vi "build.stepElement.vi"(11 "Step in":T1) -> (0 "error out":errorcluster, 3 "steps out":variant[](array[variant])=[variant("stepDoutString"=variant(string ""), "stepFunction"=variant(enum16{"__NO-OP", "_DELAY_LOAD", "_DELAY_COMPARE", "_COMPARE", "_JUMP", "_FINISH", "CLK_COMPARE", "PROC_START", "PROC_STOP", "PROC_ISRUN_IF_OFF", "PROC_ISRUN_LOAD", "_IO_READ_IN", "_IO_WRITE_DOUT", "_IO_COMPARE", "Q_OPEN", "Q_WRITE", "Q_READ"} enum."_IO_WRITE_DOUT"), "stepIoPointer"=variant(string ""), "stepLabel"=variant(string ""), "stepPath"=variant(string ""))])   [LabVIEW 2024]
uses:
  controls/UiStepBuilder.ctl
  controls/type.step-builder.ctl
  Polymorphics/variantCtrlStepFunction.vi
  Polymorphics/variantCtrlSetpoint.vi
  Polymorphics/variantCtrlString.vi
  util.DelimitedStringFromArray.vi
  Polymorphics/variantCtrlNumber.vi
  util.DelimitedStringToArray.vi
  proc.util.validateParamExist.vi
  <vilib>/Utility/error.llb/Clear Errors.vi
  <vilib>/Utility/error.llb/Trim Whitespace.vi
  <vilib>/Utility/error.llb/Trim Whitespace One-Sided.vi
  build.elementToParamString.vi
  util.error.create.vi
  Polymorphics/variantCtrlStepPointer.vi
  Polymorphics/variantCtrlStepUserMessage.vi
  Polymorphics/variantCtrlStepPath.vi
  controls/typeStepVarients.ctl
  controls/type.StepFunction.ctl
  <vilib>/Utility/miscctls.llb/LVPointTypeDef.ctl
panel:
  out "Step Argument Names":string
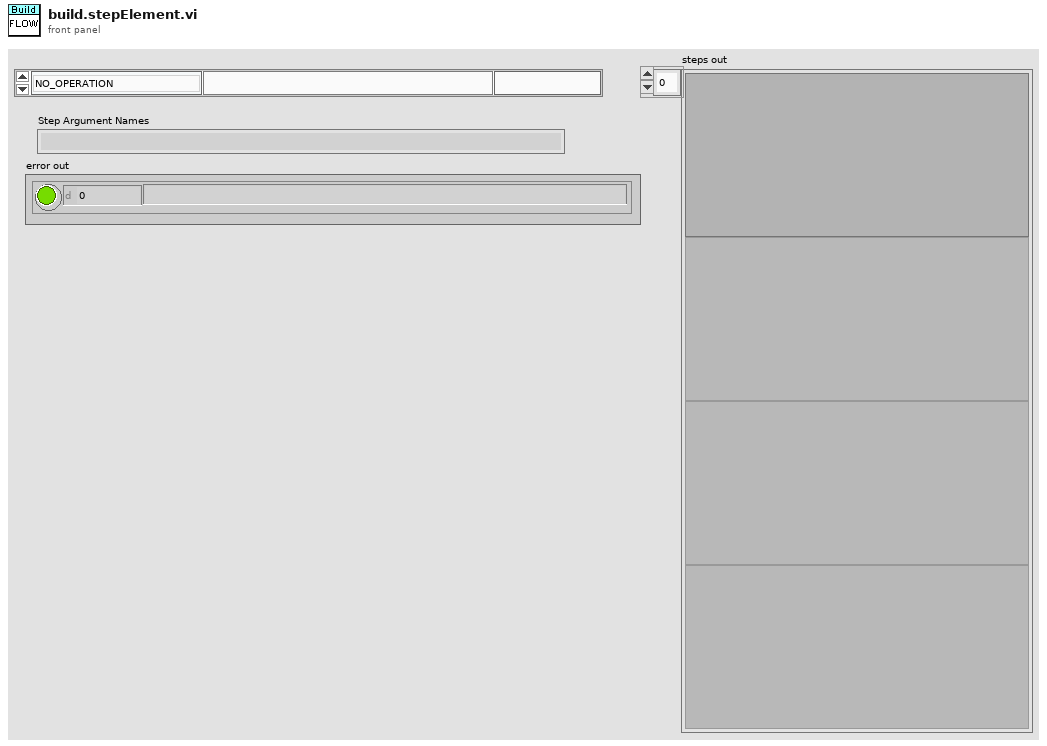
[diagram p1: front panel]
types:
  T1 = typedef "UiStepBuilder.ctl" = cluster{"Step Function":T2, "ParamString":string, "Step Label":string}
  T2 = typedef "type.step-builder.ctl" = enum16{"NO_OPERATION", "DELAY-JUMP", "DELAY", "JUMP", "COMPLETE", "SCHEDULER", "IRR-CHECK", "UNIT-CHECK", "UNIT-SAMPLE", "UNIT-DOSE", "LOG-REPORT", "LOG-MESSAGE", "IO-READ", "IO-READ-MANY", "IO-WRITE", "IO-COMPARE-OUT", "IO-COMPARE-IN", "PROC-START", "PROC-STOP", "PROC-LOAD", "PROC-IS-COMPLETED", "RECORD-MOVE", "GET-RH", "GET-UV", "GET-WD", "GET-WS", "OCS-CHECK", "OCS-RECORD"}
  T3 = cluster{"UiStepFunction":T2, "parameters string":string, "Step Label":string}
  T4 = typedef "LVPointTypeDef.ctl" = cluster{"Horizontal":i16, "Vertical":i16}
  T5 = typedef "typeStepVarients.ctl" = enum16{"stepNameID", "stepFunction", "stepReport", "stepSetpoint", "stepPointer", "stepProcPointer", "stepIoPointer", "stepIoValue", "stepFilePointer", "stepMessage", "stepTimeString", "stepNumReg", "stepStrReg", "stepSeconds", "stepUnitDoseParams", "stepUnitIndex"}
  T6 = typedef "type.StepFunction.ctl" = enum16{"__NO-OP", "_DELAY_LOAD", "_DELAY_COMPARE", "_JUMP", "_COMPLETE", "_COMPARE", "_LOG_MESSAGE", "_LOG_LAST_REPORT", "_SCHEDULE", "_SCHED_DAILY", "CLK_COMPARE", "PROC_START", "PROC_STOP", "PROC_LOAD", "PROC_COMPLETION_CHECK", "PROC_COMPLETION_LOAD", "_IO_READ", "_IO_READ_MANY", "_IO_WRITE", "_IO_WRITE_BY_REG", "_IO_GET_OUTPUT", "_OCS_CHECK", "_OCS_RECORD", "_GET_RH", "_GET_ACC_UV", "_GET_WD", "_GET_WS", "_REC_DELETE", "_REC_MOVE", "_REC_COPY", "_IRR_CHECK", "UNIT_CHECK", "UNIT_SAMPLE", "UNIT_DOSE"}
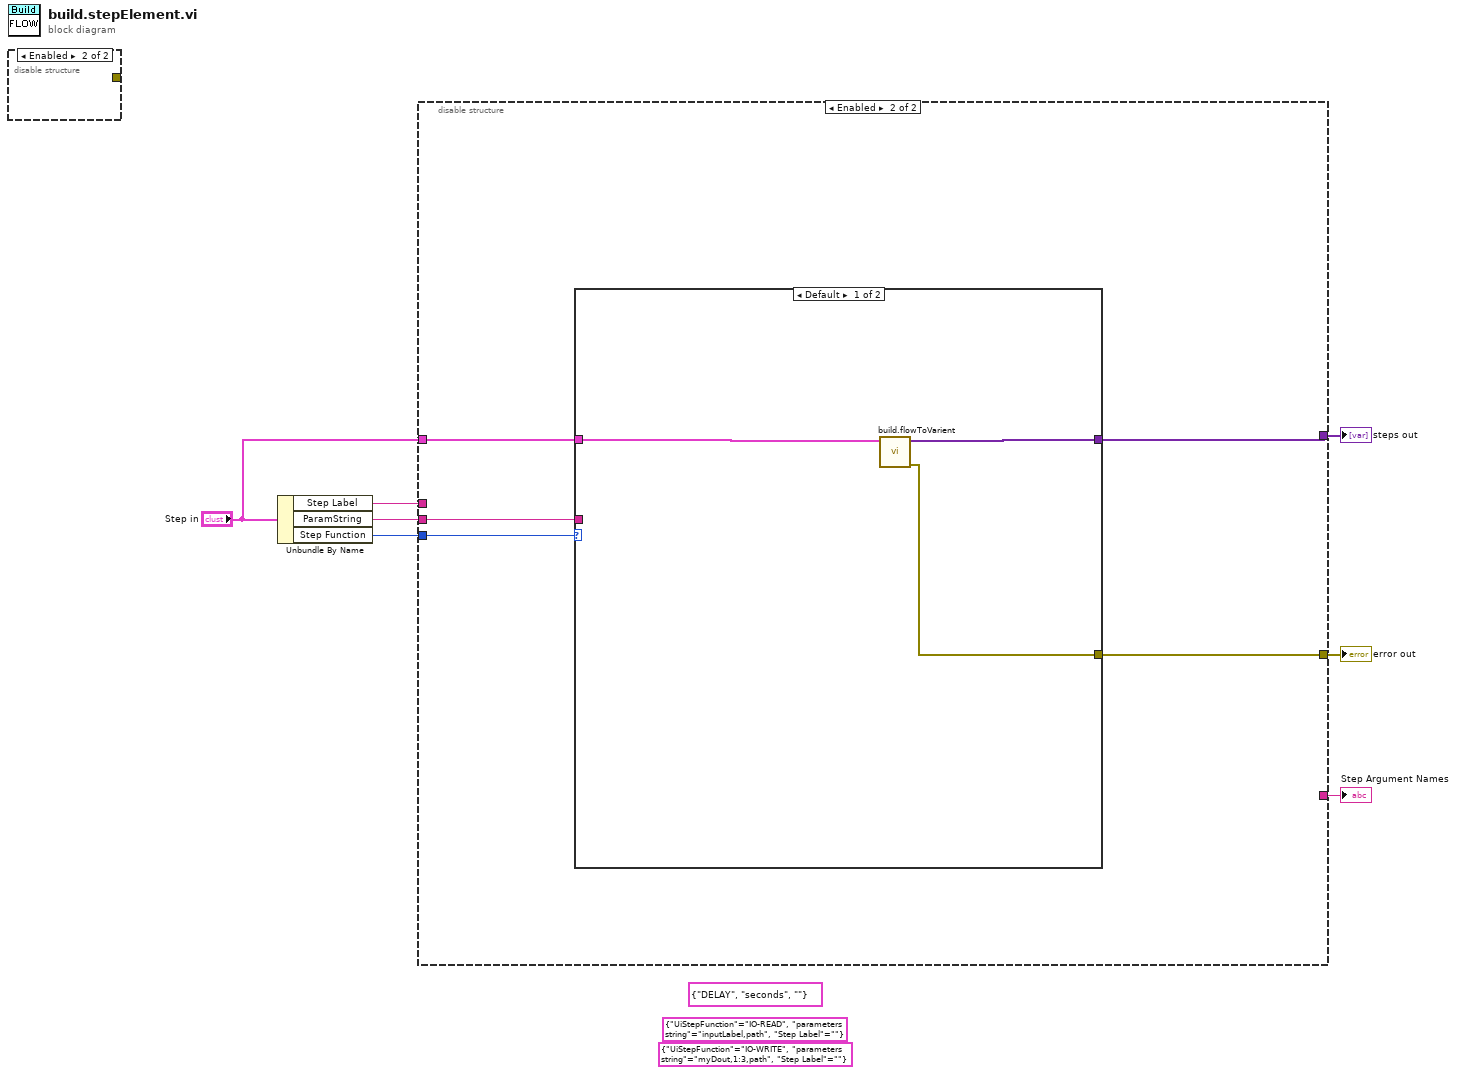
[diagram p0: block diagram]
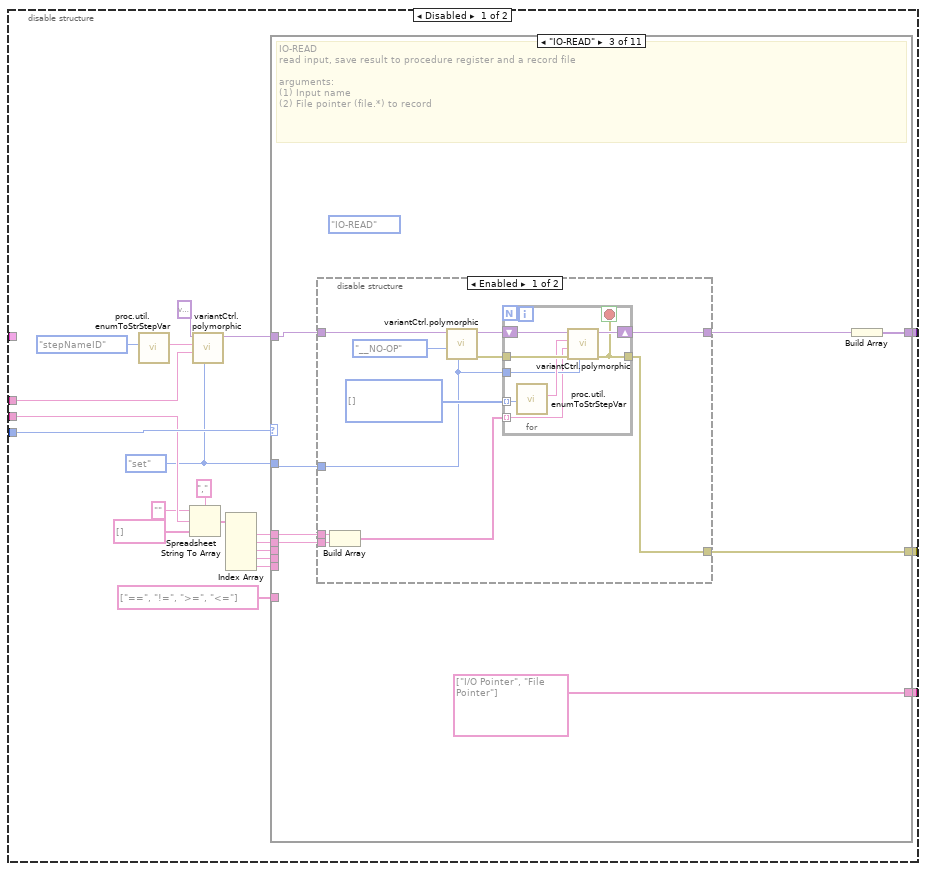
[diagram p2: hidden frame]
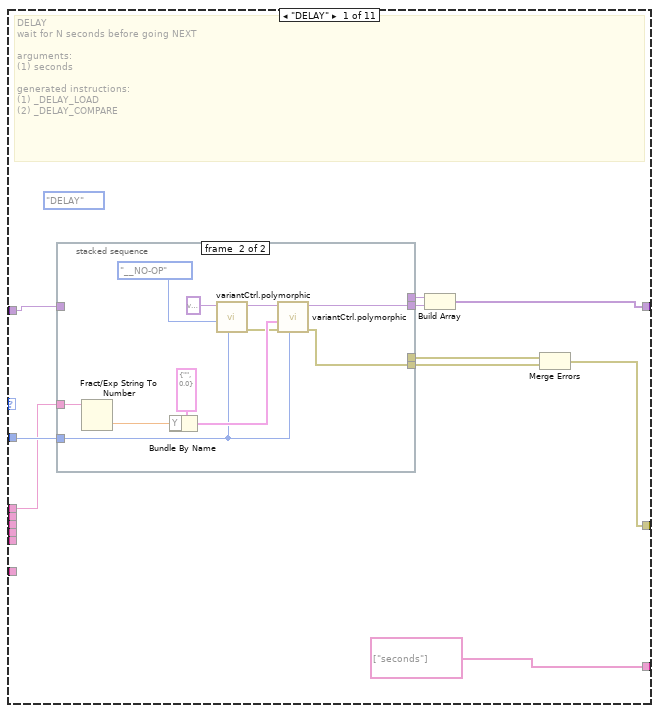
[diagram p3: hidden frame]
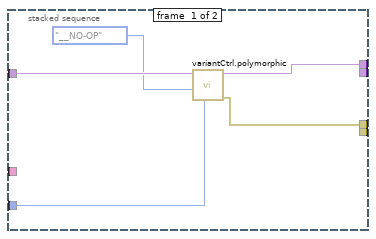
[diagram p4: hidden frame]
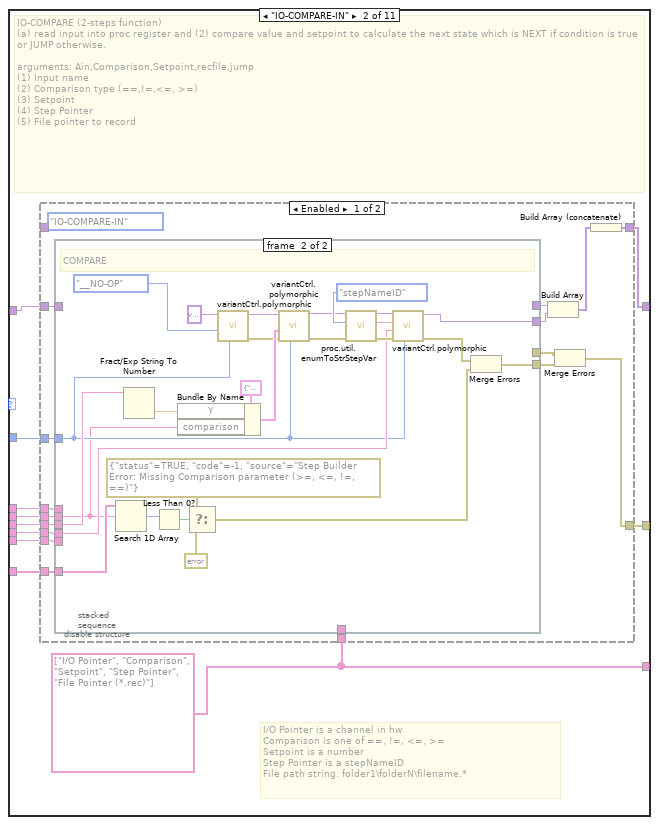
[diagram p5: hidden frame]
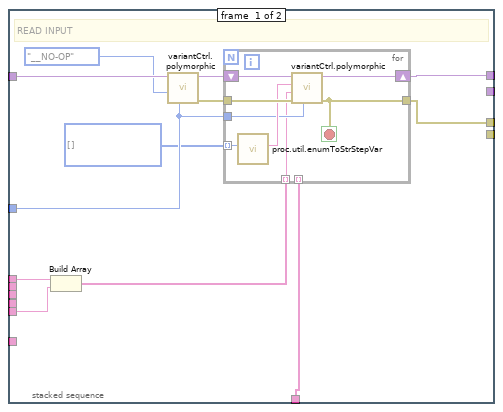
[diagram p6: hidden frame]
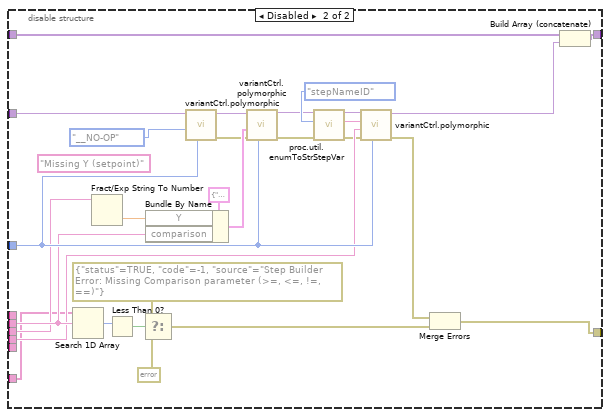
[diagram p7: hidden frame]
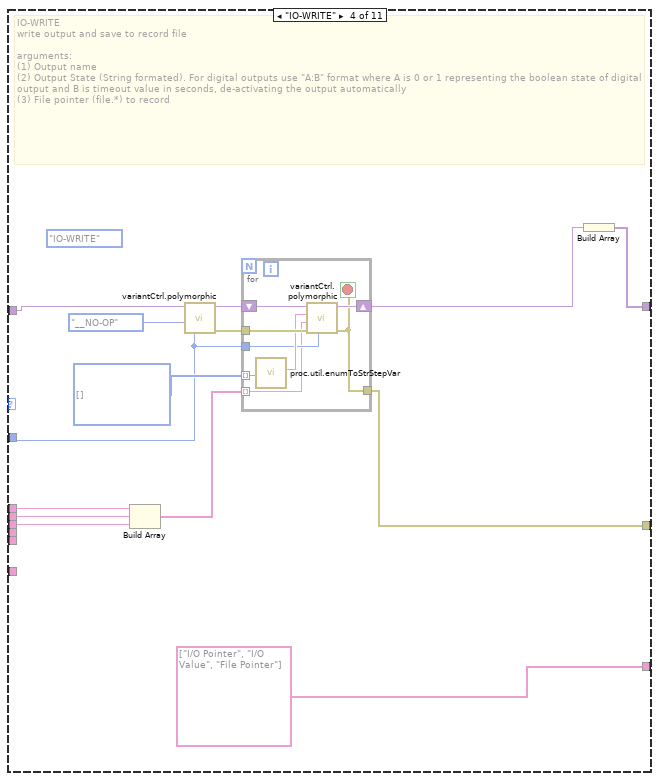
[diagram p9: hidden frame]
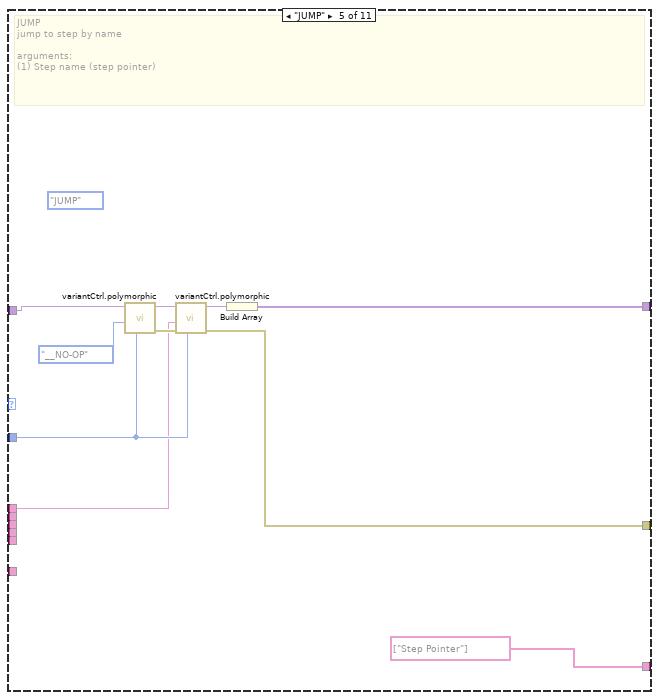
[diagram p10: hidden frame]
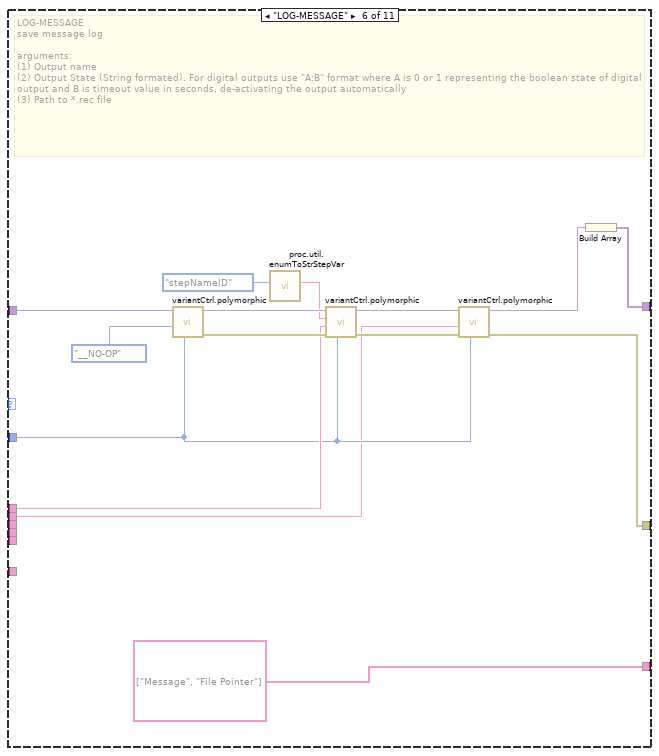
[diagram p11: hidden frame]
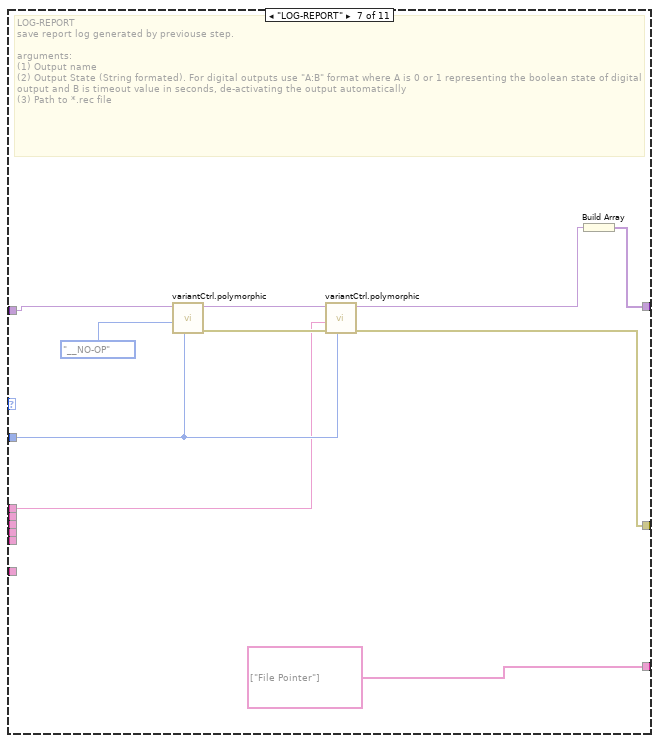
[diagram p12: hidden frame]
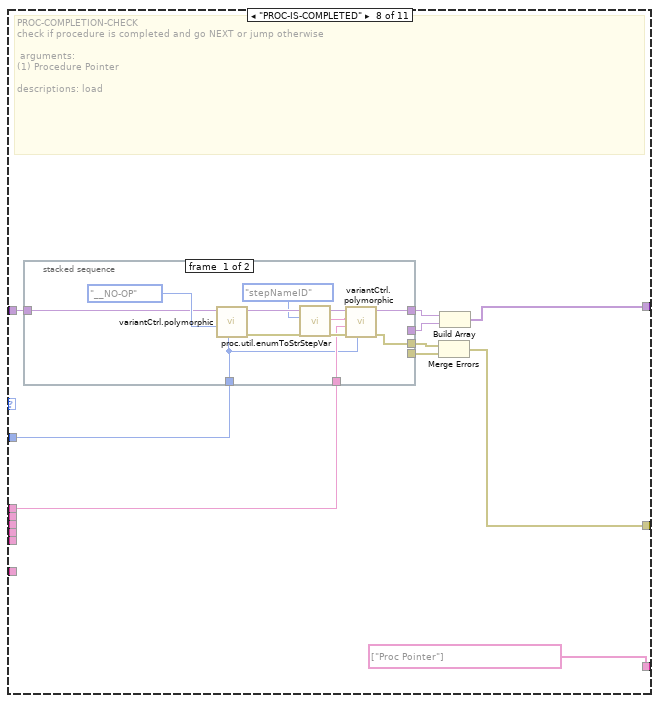
[diagram p13: hidden frame]
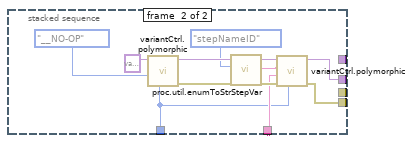
[diagram p14: hidden frame]
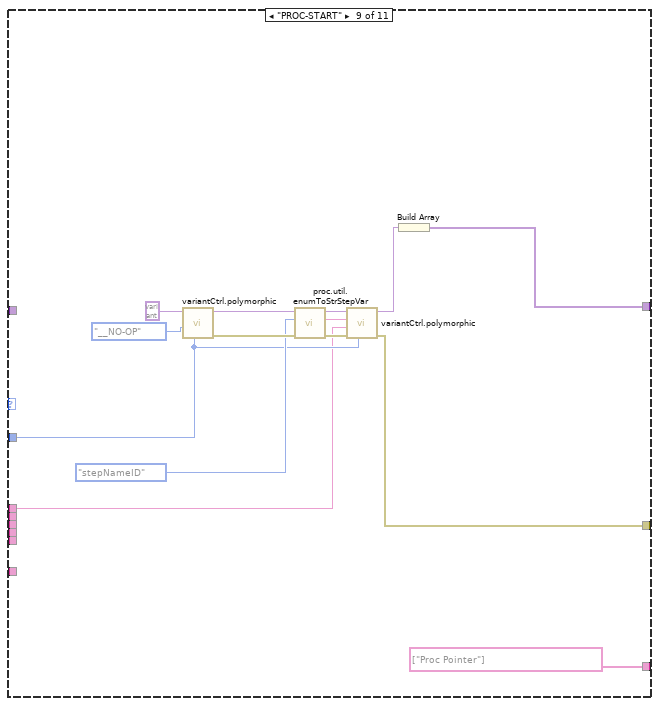
[diagram p15: hidden frame]
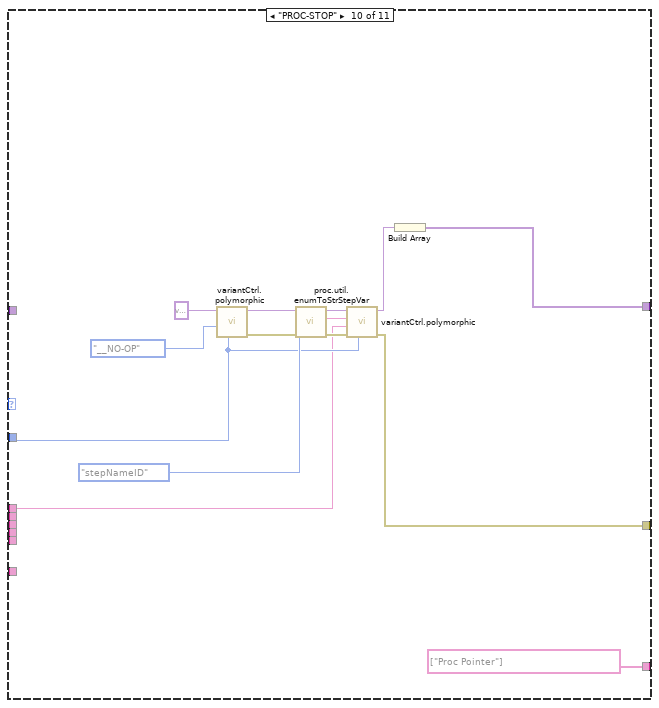
[diagram p16: hidden frame]
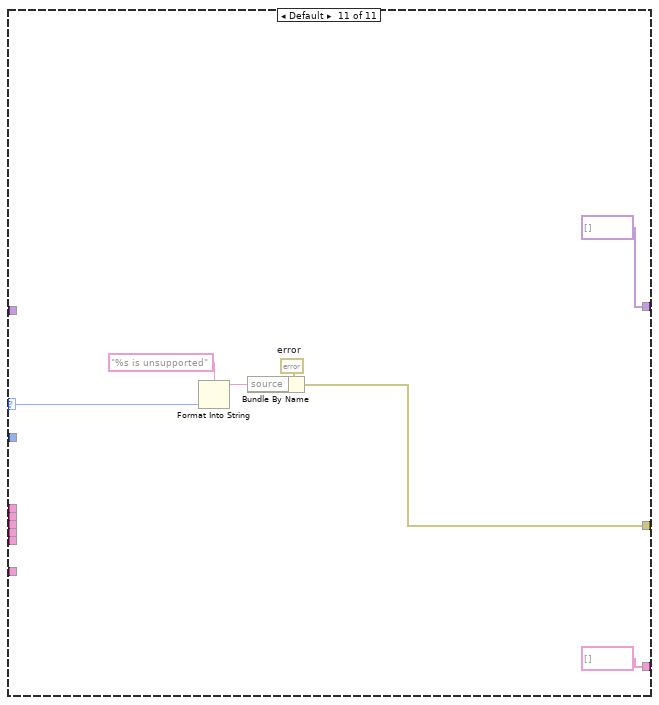
[diagram p17: hidden frame]
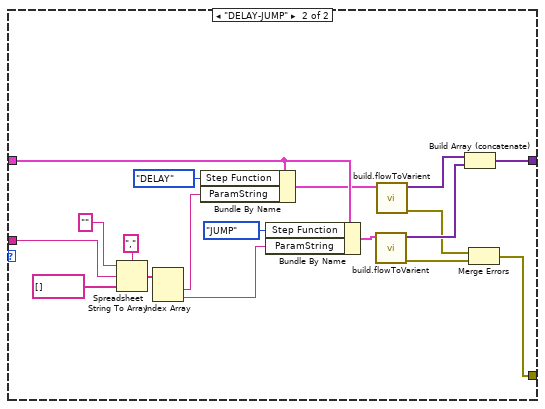
[diagram p18: hidden frame]
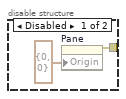
[diagram p19: hidden frame]
diagram:
  (unwired) T3 {"UiStepFunction"=enum."DELAY", "parameters string"="seconds", "Step Label"=""} ("Example DELAY Parameter String Format: seconds")
  (unwired) T3 {"UiStepFunction"=enum."IO-WRITE", "parameters string"="myDout,1:3,path", "Step Label"=""} ("Example IO-SET-DOUT Parameter String Format: IoLabel,Value:TimoutSeconds,pathToLogFile")
  (unwired) T3 {"UiStepFunction"=enum."IO-READ", "parameters string"="inputLabel,path", "Step Label"=""} ("Example IO-GET-DIN/AIN Parameter String Format: IoLabel,pathToLogFile")
  n1 = disable-structure shown="Enabled" {
    disable-tunnel: [w8 _] -> _
    frame Disabled {
      n2 = property on="Pane" class="Pane"("Origin"=T4 {"Horizontal"=0, "Vertical"=0}) -> (error out=w8:errorcluster)  [unwired: 2 in, 1 out]
    }
    frame Enabled {
    }
  }
  n3 = Unbundle By Name("Step in") -> ("Step Label"=w4:string, "ParamString"=w3:string, "Step Function"=w5:T2)
  n4 = disable-structure shown="Enabled" {
    disable-tunnel: [w30 w302] -> w7
    disable-tunnel: [w29 w301] -> w6
    disable-tunnel: w5 -> [w28 w300]
    disable-tunnel: w4 -> [w27 _]
    disable-tunnel: w3 -> [w25 w299]
    disable-tunnel: [w24 _] -> w2
    disable-tunnel: "Step in" -> [_ w303]
    frame Disabled {
      w14 = enum16{"get", "set"}."set" ("get/set")
      n5 = call "proc.util.enumToStrStepVar.vi"("Step var"=typeStepVarients."stepNameID") -> ("String"=w22:string)  [unwired: 10 in]
      n6 = Spreadsheet String To Array(delimiter (Tab)=",", format string="" ("delimiter (Tab)"), spreadsheet string=w25, array type (2D Dbl)=string[] []) -> (array=w17:string[])
      n7 = call-poly "variantCtrl.polymorphic.vi"("menu in (get)"=w14, "String Value"=w27, "name in"=w22, "Step in"=variant ("stepElement _DELAY_LOAD")) -> ("Step out"=w21:variant)  [unwired: 4 in, 3 out]
      n8 = Index Array(array=w17) -> (element #1=w16:string, element #2=w15:string, element #3=w13:string, element #4=w12:string, element #5=w11:string)  [unwired: 5 in]
      n9 = case shown="\"IO-READ\"" w28 {
        selector: w28 -> [_ _ _ _ _ _ _ _ _ _ w297]
        tunnel: [w32 w67 w161 w194 w212 w227 w237 w247 w279 w291 variant[] []] -> w30
        tunnel: [w36 w66 w160 w189 w205 w215 w233 w242 w272 w283 w294] -> w29
        tunnel: w21 -> [w35 w65 w157 w186 w208 w226 w236 w241 _ _ _]
        tunnel: w14 -> [w34 w64 w159 w188 w207 w214 w235 w240 w271 w282 _]
        tunnel: w16 -> [w33 w63 w158 w187 w204 w221 w229 w239 w269 w281 _]
        tunnel: w15 -> [_ w62 w155 w182 _ w213 _ _ _ _ _]
        tunnel: w13 -> [_ w61 _ w183 _ _ _ _ _ _ _]
        tunnel: w12 -> [_ w60 _ _ _ _ _ _ _ _ _]
        tunnel: w11 -> [_ w59 _ _ _ _ _ _ _ _ _]
        tunnel: string[] ["==", "!=", ">=", "<="] ("source") -> [_ w58 _ _ _ _ _ _ _ _ _]
        tunnel: [string[] ["seconds"] ("source") w57 string[] ["I/O Pointer", "File Pointer"] ("source") string[] ["I/O Pointer", "I/O Value", "File Pointer"] ("source") string[] ["Step Pointer"] ("source") string[] ["Message", "File Pointer"] ("source") string[] ["File Pointer"] ("source") string[] ["Proc Pointer"] ("source") string[] ["Proc Pointer"] ("source") string[] ["Proc Pointer"] ("source") string[] [] ("source")] -> w24
        frame "DELAY" {
          (unwired) type.step-builder."DELAY" ("UiStepFunction")
          # "DELAY\nwait for N seconds before going NEXT\n\narguments:\n(1) seconds\n\ngenerated instructions:\n(1) _DELAY_LOAD\n(2) _DELAY_COMPARE"
          n10 = stacked-sequence {
            tunnel: [w43 _] -> w40
            tunnel: [_ w47] -> w39
            tunnel: [_ w55] -> w38
            tunnel: [w42 _] -> w37
            tunnel: w33 -> [_ w54]
            tunnel: w35 -> [w45 _]
            tunnel: w34 -> [w44 w50]
            frame #0 {
              n11 = call-poly "variantCtrl.polymorphic.vi"("menu in (get)"=w44, "StepFunction"=type.StepFunction."__NO-OP" ("Operation out"), "variant in"=w45) -> ("error out"=w42:errorcluster, "variant out"=w43:variant)  [unwired: 5 in, 2 out]
            }
            frame #1 {
              n12 = Fract/Exp String To Number(string=w54) -> (number=w53:dbl)  [unwired: 3 in, 1 out]
              n13 = Bundle By Name(cluster=cluster{"comparison":string, "Y":dbl} {"comparison"="", "Y"=0.0} ("setpoint 2"), "Y"=w53) -> (w56:cluster{"comparison":string, "Y":dbl})
              n14 = call-poly "variantCtrl.polymorphic.vi"("menu in (get)"=w50, "StepFunction"=type.StepFunction."__NO-OP" ("Operation out"), "variant in"=variant ("stepElement _DELAY_LOAD")) -> ("error out"=w51:errorcluster, "variant out"=w52:variant)  [unwired: 5 in, 2 out]
              n15 = call-poly "variantCtrl.polymorphic.vi"("get/set"=w50, "error in"=w51, "setpoint"=w56, "procElement in in"=w52) -> ("error out"=w55:errorcluster, "procElement out"=w47:variant)  [unwired: 4 in, 2 out]
            }
          }
          n16 = Build Array(w40, w39) -> (w32:variant[])
          n17 = Merge Errors(w37, w38) -> (w36:errorcluster)
        }
        frame "IO-COMPARE-IN" {
          w57 = string[] ["I/O Pointer", "Comparison", "Setpoint", "Step Pointer", "File Pointer (*.rec)"] ("source")
          # "I/O Pointer is a channel in hw \nComparison is one of ==, !=, <=, >=\nSetpoint is a number\nStep Pointer is a stepNameID\nFile path string. folder1\\folderN\\filename.*"
          # "IO-COMPARE (2-steps function)\n(a) read input into proc register and (2) compare value and setpoint to calculate the next state which is NEXT if condition is true or JUMP otherwise. \n\narguments: Ain,Comparison,Setpoint,recfile,jump\n(1) Input name\n(2) Comparison type (==,!=,<=, >=)\n(3) Setpoint\n(4) Step Pointer\n(5) File pointer to record"
          n18 = disable-structure shown="Enabled" {
            disable-tunnel: _ -> [_ w153]
            disable-tunnel: [w83 w152] -> w67
            disable-tunnel: [w81 w129] -> w66
            disable-tunnel: w65 -> [w80 w128]
            disable-tunnel: w64 -> [w79 w151]
            disable-tunnel: w63 -> [w78 _]
            disable-tunnel: w62 -> [w77 w150]
            disable-tunnel: w61 -> [w75 w149]
            disable-tunnel: w60 -> [w74 w148]
            disable-tunnel: w59 -> [w73 _]
            disable-tunnel: w58 -> [w72 w147]
            disable-tunnel: w57 -> [w68 _]
            frame Enabled {
              (unwired) type.step-builder."IO-COMPARE-IN" ("UiStepFunction")
              n19 = stacked-sequence {
                tunnel: [w92 _] -> w82
                tunnel: w78 -> [w93 _]
                tunnel: w80 -> [w95 _]
                tunnel: w79 -> [w94 w111]
                tunnel: w77 -> [_ w109]
                tunnel: w75 -> [_ w120]
                tunnel: w74 -> [_ w112]
                tunnel: w73 -> [w85 _]
                tunnel: w72 -> [_ w110]
                tunnel: [_ w105] -> w71
                tunnel: [w86 _] -> w70
                tunnel: [_ w104] -> w69
                tunnel: w68 -> [w84 _]
                frame #0 {
                  w88 = T5[] [] items=["stepNameID", "stepFunction", "stepReport", "stepSetpoint", "stepPointer", "stepProcPointer", "stepIoPointer", "stepIoValue", "stepFilePointer", "stepMessage", "stepTimeString", "stepNumReg", "stepStrReg", "stepSeconds", "stepUnitDoseParams", "stepUnitIndex"] ("Step var")
                  # "READ INPUT"
                  n20 = Build Array(w93, w85) -> (w87:string[])
                  n21 = call-poly "variantCtrl.polymorphic.vi"("menu in (get)"=w94, "StepFunction"=type.StepFunction."__NO-OP" ("Operation out"), "variant in"=w95) -> ("error out"=w91:errorcluster, "variant out"=w90:variant)  [unwired: 5 in, 2 out]
                  n22 = for {
                    tunnel: w88 -> [w101] mode=indexing
                    tunnel: w94 -> [w99]
                    tunnel: w87 -> [w98] mode=indexing
                    shift-right: [w97] -> w86
                    shift-left: w90 -> [w102]
                    tunnel: w91 -> [w103]
                    tunnel: [w96] -> w92
                    tunnel: w84 -> [_] mode=indexing
                    stop <- w96 stop-if-true
                    n23 = call "proc.util.enumToStrStepVar.vi"("Step var"=w101) -> ("String"=w100:string)  [unwired: 10 in]
                    n24 = call-poly "variantCtrl.polymorphic.vi"("menu in (get)"=w99, "error in"=w103, "String Value"=w98, "name in"=w100, "Step in"=w102) -> ("error out"=w96:errorcluster, "Step out"=w97:variant)  [unwired: 3 in, 2 out]
                  }
                }
                frame #1 {
                  # "COMPARE"
                  n25 = Search 1D Array(1D array=w110, element=w109) -> (index of element=w108:i32)  [unwired: 1 in]
                  n26 = Fract/Exp String To Number(string=w120) -> (number=w125:dbl)  [unwired: 3 in, 1 out]
                  n27 = Less Than 0?(x=w108) -> (x < 0?=w107:bool)
                  n28 = Bundle By Name(cluster=cluster{"comparison":string, "Y":dbl} {"comparison"="", "Y"=0.0} ("setpoint"), "Y"=w125, "comparison"=w109) -> (w127:cluster{"comparison":string, "Y":dbl})
                  n29 = Select(t=errorcluster {"status"=TRUE, "code"=-1, "source"="Step Builder Error: Missing Comparison parameter (>=, <=, !=, ==)"} ("error out"), s=w107, f=errorcluster {"status"=FALSE, "code"=0, "source"=""}) -> (s? t:f=w118:errorcluster)
                  n30 = call-poly "variantCtrl.polymorphic.vi"("menu in (get)"=w111, "StepFunction"=type.StepFunction."__NO-OP" ("Operation out"), "variant in"=variant ("stepElement _DELAY_LOAD")) -> ("error out"=w123:errorcluster, "variant out"=w124:variant)  [unwired: 5 in, 2 out]
                  n31 = call-poly "variantCtrl.polymorphic.vi"("get/set"=w111, "error in"=w123, "setpoint"=w127, "procElement in in"=w124) -> ("error out"=w113:errorcluster, "procElement out"=w115:variant)  [unwired: 4 in, 2 out]
                  n32 = call "proc.util.enumToStrStepVar.vi"("Step var"=typeStepVarients."stepNameID") -> ("String"=w116:string)  [unwired: 10 in]
                  n33 = call-poly "variantCtrl.polymorphic.vi"("menu in (get)"=w111, "error in"=w113, "String Value"=w112, "name in"=w116, "Step in"=w115) -> ("error out"=w114:errorcluster, "Step out"=w105:variant)  [unwired: 3 in, 2 out]
                  n34 = Merge Errors(w114, w118) -> (w104:errorcluster)
                }
              }
              n35 = Build Array(w70, w71) -> (w76:variant[])
              n36 = Merge Errors(w82, w69) -> (w81:errorcluster)
              n37 = Build Array (concatenate)(w76) -> (w83:variant[])
            }
            frame Disabled {
              (unwired) "Missing Y (setpoint)" ("delimiter (Tab)")
              n38 = Search 1D Array(1D array=w147, element=w150) -> (index of element=w132:i32)  [unwired: 1 in]
              n39 = Fract/Exp String To Number(string=w149) -> (number=w143:dbl)  [unwired: 3 in, 1 out]
              n40 = Less Than 0?(x=w132) -> (x < 0?=w131:bool)
              n41 = Select(t=errorcluster {"status"=TRUE, "code"=-1, "source"="Step Builder Error: Missing Comparison parameter (>=, <=, !=, ==)"} ("error out"), s=w131, f=errorcluster {"status"=FALSE, "code"=0, "source"=""}) -> (s? t:f=w138:errorcluster)
              n42 = Bundle By Name(cluster=cluster{"comparison":string, "Y":dbl} {"comparison"="", "Y"=0.0} ("setpoint"), "Y"=w143, "comparison"=w150) -> (w145:cluster{"comparison":string, "Y":dbl})
              n43 = call-poly "variantCtrl.polymorphic.vi"("menu in (get)"=w151, "StepFunction"=type.StepFunction."__NO-OP" ("Operation out"), "variant in"=w128) -> ("error out"=w141:errorcluster, "variant out"=w142:variant)  [unwired: 5 in, 2 out]
              n44 = call-poly "variantCtrl.polymorphic.vi"("get/set"=w151, "error in"=w141, "setpoint"=w145, "procElement in in"=w142) -> ("error out"=w133:errorcluster, "procElement out"=w135:variant)  [unwired: 4 in, 2 out]
              n45 = call "proc.util.enumToStrStepVar.vi"("Step var"=typeStepVarients."stepNameID") -> ("String"=w136:string)  [unwired: 10 in]
              n46 = call-poly "variantCtrl.polymorphic.vi"("menu in (get)"=w151, "error in"=w133, "String Value"=w148, "name in"=w136, "Step in"=w135) -> ("error out"=w134:errorcluster, "Step out"=w146:variant)  [unwired: 3 in, 2 out]
              n47 = Merge Errors(w134, w138) -> (w129:errorcluster)
              n48 = Build Array (concatenate)(w153, w146) -> (w152:variant[])
            }
          }
        }
        frame "IO-READ" {
          (unwired) type.step-builder."IO-READ" ("UiStepFunction")
          # "IO-READ\nread input, save result to procedure register and a record file\n\narguments:\n(1) Input name\n(2) File pointer (file.*) to record"
          n49 = disable-structure shown="Enabled" {
            disable-tunnel: [w168 _] -> w160
            disable-tunnel: w159 -> [w167 _]
            disable-tunnel: w158 -> [w166 _]
            disable-tunnel: w157 -> [w165 _]
            disable-tunnel: [w164 _] -> w156
            disable-tunnel: w155 -> [w162 _]
            frame Enabled {
              w169 = T5[] [] items=["stepNameID", "stepFunction", "stepReport", "stepSetpoint", "stepPointer", "stepProcPointer", "stepIoPointer", "stepIoValue", "stepFilePointer", "stepMessage", "stepTimeString", "stepNumReg", "stepStrReg", "stepSeconds", "stepUnitDoseParams", "stepUnitIndex"] ("Step var")
              n50 = Build Array(w166, w162) -> (w163:string[])
              n51 = call-poly "variantCtrl.polymorphic.vi"("menu in (get)"=w167, "StepFunction"=type.StepFunction."__NO-OP" ("Operation out"), "variant in"=w165) -> ("error out"=w172:errorcluster, "variant out"=w171:variant)  [unwired: 5 in, 2 out]
              n52 = for {
                tunnel: w169 -> [w178] mode=indexing
                tunnel: w167 -> [w176]
                tunnel: w163 -> [w175] mode=indexing
                shift-right: [w174] -> w164
                shift-left: w171 -> [w179]
                tunnel: w172 -> [w180]
                tunnel: [w173] -> w168
                stop <- w173 stop-if-true
                n53 = call "proc.util.enumToStrStepVar.vi"("Step var"=w178) -> ("String"=w177:string)  [unwired: 10 in]
                n54 = call-poly "variantCtrl.polymorphic.vi"("menu in (get)"=w176, "error in"=w180, "String Value"=w175, "name in"=w177, "Step in"=w179) -> ("error out"=w173:errorcluster, "Step out"=w174:variant)  [unwired: 3 in, 2 out]
              }
            }
            frame Disabled {
            }
          }
          n55 = Build Array(w156) -> (w161:variant[])
        }
        frame "IO-WRITE" {
          (unwired) type.step-builder."IO-WRITE" ("UiStepFunction")
          w190 = T5[] [] items=["stepNameID", "stepFunction", "stepReport", "stepSetpoint", "stepPointer", "stepProcPointer", "stepIoPointer", "stepIoValue", "stepFilePointer", "stepMessage", "stepTimeString", "stepNumReg", "stepStrReg", "stepSeconds", "stepUnitDoseParams", "stepUnitIndex"] ("Step var")
          # "IO-WRITE\nwrite output and save to record file\n\narguments:\n(1) Output name\n(2) Output State (String formated). For digital outputs use \"A:B\" format where A is 0 or 1 representing the boolean state of digital output and B is timeout value in seconds, de-activating the output automatically\n(3) File pointer (file.*) to record"
          n56 = Build Array(w187, w182, w183) -> (w184:string[])
          n57 = call-poly "variantCtrl.polymorphic.vi"("menu in (get)"=w188, "StepFunction"=type.StepFunction."__NO-OP" ("Operation out"), "variant in"=w186) -> ("error out"=w193:errorcluster, "variant out"=w192:variant)  [unwired: 5 in, 2 out]
          n58 = for {
            tunnel: w190 -> [w200] mode=indexing
            tunnel: w188 -> [w198]
            tunnel: w184 -> [w197] mode=indexing
            shift-right: [w196] -> w185
            shift-left: w192 -> [w201]
            tunnel: w193 -> [w202]
            tunnel: [w195] -> w189
            stop <- w195 stop-if-true
            n59 = call "proc.util.enumToStrStepVar.vi"("Step var"=w200) -> ("String"=w199:string)  [unwired: 10 in]
            n60 = call-poly "variantCtrl.polymorphic.vi"("menu in (get)"=w198, "error in"=w202, "String Value"=w197, "name in"=w199, "Step in"=w201) -> ("error out"=w195:errorcluster, "Step out"=w196:variant)  [unwired: 3 in, 2 out]
          }
          n61 = Build Array(w185) -> (w194:variant[])
        }
        frame "JUMP" {
          (unwired) type.step-builder."JUMP" ("UiStepFunction")
          # "JUMP\njump to step by name\n\narguments:\n(1) Step name (step pointer)"
          n62 = call-poly "variantCtrl.polymorphic.vi"("menu in (get)"=w207, "StepFunction"=type.StepFunction."__NO-OP" ("Operation out"), "variant in"=w208) -> ("error out"=w209:errorcluster, "variant out"=w210:variant)  [unwired: 5 in, 2 out]
          n63 = call-poly "variantCtrl.polymorphic.vi"("menu in (get)"=w207, "error in"=w209, "String in"=w204, "stepElement in in"=w210) -> ("error out"=w205:errorcluster, "stepElement out"=w206:variant)  [unwired: 4 in, 2 out]
          n64 = Build Array(w206) -> (w212:variant[])
        }
        frame "LOG-MESSAGE" {
          # "LOG-MESSAGE\nsave message log\n \narguments:\n(1) Output name\n(2) Output State (String formated). For digital outputs use \"A:B\" format where A is 0 or 1 representing the boolean state of digital output and B is timeout value in seconds, de-activating the output automatically\n(3) Path to *.rec file"
          n65 = call-poly "variantCtrl.polymorphic.vi"("menu in (get)"=w214, "StepFunction"=type.StepFunction."__NO-OP" ("Operation out"), "variant in"=w226) -> ("error out"=w223:errorcluster, "variant out"=w224:variant)  [unwired: 5 in, 2 out]
          n66 = call "proc.util.enumToStrStepVar.vi"("Step var"=typeStepVarients."stepNameID") -> ("String"=w220:string)  [unwired: 10 in]
          n67 = call-poly "variantCtrl.polymorphic.vi"("menu in (get)"=w214, "error in"=w223, "String Value"=w221, "name in"=w220, "Step in"=w224) -> ("error out"=w216:errorcluster, "Step out"=w218:variant)  [unwired: 3 in, 2 out]
          n68 = call-poly "variantCtrl.polymorphic.vi"("menu(get)"=w214, "error in (no error)"=w216, "File Pointer in"=w213, "stepElement in"=w218) -> ("error out"=w215:errorcluster, "step\\element out"=w217:variant)  [unwired: 5 in, 1 out]
          n69 = Build Array(w217) -> (w227:variant[])
        }
        frame "LOG-REPORT" {
          # "LOG-REPORT\nsave report log generated by previouse step.\n\narguments:\n(1) Output name\n(2) Output State (String formated). For digital outputs use \"A:B\" format where A is 0 or 1 representing the boolean state of digital output and B is timeout value in seconds, de-activating the output automatically\n(3) Path to *.rec file"
          n70 = call-poly "variantCtrl.polymorphic.vi"("menu in (get)"=w235, "StepFunction"=type.StepFunction."__NO-OP" ("Operation out"), "variant in"=w236) -> ("error out"=w230:errorcluster, "variant out"=w231:variant)  [unwired: 5 in, 2 out]
          n71 = call-poly "variantCtrl.polymorphic.vi"("menu(get)"=w235, "error in (no error)"=w230, "File Pointer in"=w229, "stepElement in"=w231) -> ("error out"=w233:errorcluster, "step\\element out"=w234:variant)  [unwired: 5 in, 1 out]
          n72 = Build Array(w234) -> (w237:variant[])
        }
        frame "PROC-IS-COMPLETED" {
          # "PROC-COMPLETION-CHECK \ncheck if procedure is completed and go NEXT or jump otherwise\n\n arguments:\n(1) Procedure Pointer\n\ndescriptions: load"
          n73 = stacked-sequence {
            tunnel: [w254 _] -> w246
            tunnel: [_ w262] -> w245
            tunnel: w239 -> [w251 w261]
            tunnel: [w250 _] -> w244
            tunnel: [_ w260] -> w243
            tunnel: w241 -> [w249 _]
            tunnel: w240 -> [w248 w259]
            frame #0 {
              n74 = call-poly "variantCtrl.polymorphic.vi"("menu in (get)"=w248, "StepFunction"=type.StepFunction."__NO-OP" ("Operation out"), "variant in"=w249) -> ("error out"=w257:errorcluster, "variant out"=w256:variant)  [unwired: 5 in, 2 out]
              n75 = call "proc.util.enumToStrStepVar.vi"("Step var"=typeStepVarients."stepNameID") -> ("String"=w253:string)  [unwired: 10 in]
              n76 = call-poly "variantCtrl.polymorphic.vi"("menu in (get)"=w248, "error in"=w257, "String Value"=w251, "name in"=w253, "Step in"=w256) -> ("error out"=w250:errorcluster, "Step out"=w254:variant)  [unwired: 3 in, 2 out]
            }
            frame #1 {
              n77 = call-poly "variantCtrl.polymorphic.vi"("menu in (get)"=w259, "StepFunction"=type.StepFunction."__NO-OP" ("Operation out"), "variant in"=variant) -> ("error out"=w267:errorcluster, "variant out"=w266:variant)  [unwired: 5 in, 2 out]
              n78 = call "proc.util.enumToStrStepVar.vi"("Step var"=typeStepVarients."stepNameID") -> ("String"=w264:string)  [unwired: 10 in]
              n79 = call-poly "variantCtrl.polymorphic.vi"("menu in (get)"=w259, "error in"=w267, "String Value"=w261, "name in"=w264, "Step in"=w266) -> ("error out"=w260:errorcluster, "Step out"=w262:variant)  [unwired: 3 in, 2 out]
            }
          }
          n80 = Merge Errors(w244, w243) -> (w242:errorcluster)
          n81 = Build Array(w246, w245) -> (w247:variant[])
        }
        frame "PROC-START" {
          n82 = call-poly "variantCtrl.polymorphic.vi"("menu in (get)"=w271, "StepFunction"=type.StepFunction."__NO-OP" ("Operation out"), "variant in"=variant ("stepElement")) -> ("error out"=w278:errorcluster, "variant out"=w277:variant)  [unwired: 5 in, 2 out]
          n83 = call "proc.util.enumToStrStepVar.vi"("Step var"=typeStepVarients."stepNameID") -> ("String"=w273:string)  [unwired: 10 in]
          n84 = call-poly "variantCtrl.polymorphic.vi"("menu in (get)"=w271, "error in"=w278, "String Value"=w269, "name in"=w273, "Step in"=w277) -> ("error out"=w272:errorcluster, "Step out"=w270:variant)  [unwired: 3 in, 2 out]
          n85 = Build Array(w270) -> (w279:variant[])
        }
        frame "PROC-STOP" {
          n86 = call-poly "variantCtrl.polymorphic.vi"("menu in (get)"=w282, "StepFunction"=type.StepFunction."__NO-OP" ("Operation out"), "variant in"=variant ("stepElement")) -> ("error out"=w289:errorcluster, "variant out"=w288:variant)  [unwired: 5 in, 2 out]
          n87 = call "proc.util.enumToStrStepVar.vi"("Step var"=typeStepVarients."stepNameID") -> ("String"=w284:string)  [unwired: 10 in]
          n88 = call-poly "variantCtrl.polymorphic.vi"("menu in (get)"=w282, "error in"=w289, "String Value"=w281, "name in"=w284, "Step in"=w288) -> ("error out"=w283:errorcluster, "Step out"=w290:variant)  [unwired: 3 in, 2 out]
          n89 = Build Array(w290) -> (w291:variant[])
        }
        frame Default {
          w296 = errorcluster {"status"=TRUE, "code"=-1, "source"=""}  # error
          n90 = Format Into String(format string="%s is unsupported", w297) -> (resulting string=w295:string)  [unwired: 2 in, 1 out]
          n91 = Bundle By Name(cluster=w296, "source"=w295) -> (w294:errorcluster)
        }
      }
    }
    frame Enabled {
      n92 = case shown="Default" w300 {
        tunnel: w303 -> [w306 w313]
        tunnel: [w305 w317] -> w302
        tunnel: [w304 w307] -> w301
        tunnel: w299 -> [_ w321]
        frame Default {
          n93 = call "build.flowToVarient.vi"("Flow Element"=w306) -> ("error out"=w304:errorcluster, "instructions out"=w305:variant[])  [unwired: 9 in]
        }
        frame "DELAY-JUMP" {
          n94 = Spreadsheet String To Array(delimiter (Tab)=",", format string="" ("delimiter (Tab)"), spreadsheet string=w321, array type (2D Dbl)=string[] []) -> (array=w322:string[])
          n95 = Index Array(array=w322) -> (element #1=w311:string, element #2=w310:string)  [unwired: 2 in]
          n96 = Bundle By Name(cluster=w313, "Step Function"=type.step-builder."DELAY" ("UiStepFunction"), "ParamString"=w311) -> (w312:T1)
          n97 = Bundle By Name(cluster=w313, "Step Function"=type.step-builder."JUMP" ("UiStepFunction"), "ParamString"=w310) -> (w314:T1)
          n98 = call "build.flowToVarient.vi"("Flow Element"=w314) -> ("error out"=w308:errorcluster, "instructions out"=w318:variant[])  [unwired: 9 in]
          n99 = call "build.flowToVarient.vi"("Flow Element"=w312) -> ("error out"=w309:errorcluster, "instructions out"=w319:variant[])  [unwired: 9 in]
          n100 = Build Array (concatenate)(w319, w318) -> (w317:variant[])
          n101 = Merge Errors(w309, w308) -> (w307:errorcluster)
        }
      }
    }
  }
  "error out" <- w6
  "steps out" <- w7
  "Step Argument Names" <- w2
